vi "OpenNetworkStreamWriter.vi"(6 "connection timeout":i32=-1, 7 "writer buffer size":i32, 8 "error in (no error)":errorcluster, 9 "reader url":string, 10 "writer name":string, 11 "NetworkStreamWriter in":refnum<class "NetworkStreamWriter.lvclass">) -> (0 "error out":errorcluster, 1 "Initialized?":bool, 2 "Writer Endpoint":refnum<k21>, 3 "NetworkStreamWriter out":refnum<class "NetworkStreamWriter.lvclass">)   [LabVIEW 2011, in "NetworkStreamWriter.lvclass"]
doc: "Opens a network stream writer endpoint. This VI persistently tries to open the connection until it is successful or the e-stop is triggered."
uses:
  NetworkStreamWriter.lvclass
  Shared/message.ctl
  NetworkStreamWriter.lvclass/NetworkStreamWriter.ctl
  2-Think/2 Globals/2 Global.vi
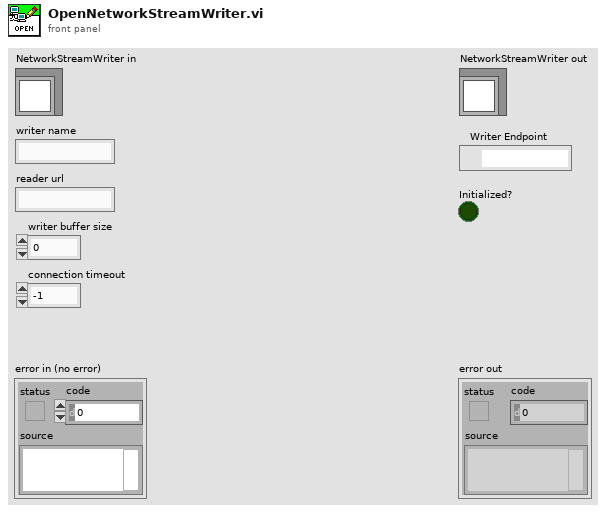
[diagram p1: front panel]
types:
  T1 = typedef "message.ctl" = cluster{"Data":variant, "Time since start (s)":dbl}
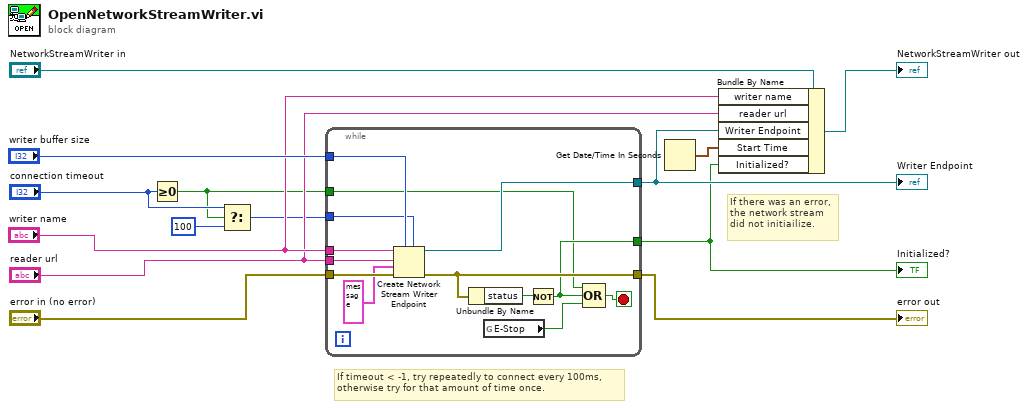
[diagram p0: block diagram]
diagram:
  # "If there was an error,\nthe network stream\ndid not initiailize."
  # "If timeout < -1, try repeatedly to connect every 100ms,\notherwise try for that amount of time once."
  n1 = Greater Or Equal To 0?(x="connection timeout") -> (x >= 0?=w3:bool)
  n2 = Select(t="connection timeout", s=w3, f=100 ("t")) -> (s? t:f=w2:i32)
  n3 = while {
    tunnel: "error in (no error)" -> [w27]
    tunnel: "writer buffer size" -> [w26]
    tunnel: [w22] -> w13
    tunnel: "writer name" -> [w25]
    tunnel: "reader url" -> [w24]
    tunnel: [w21] -> w7
    tunnel: [w18] -> w4
    tunnel: w3 -> [w16]
    tunnel: w2 -> [w15]
    stop <- w19 stop-if-true
    n4 = Create Network Stream Writer Endpoint(5:w15, 7:w26, 8:w27, 9:T1 {"Data"=variant, "Time since start (s)"=0.0} ("variant"), 10:w24, 11:w25) -> (0:w22:errorcluster, 3:w21:refnum<k21>)
    n5 = Unbundle By Name(w22) -> ("status"=w20:bool)
    n6 = global read "2 Global.vi" "E-Stop"() -> (w17:bool)
    n7 = Not(x=w20) -> (.not. x?=w18:bool)
    n8 = Compound Arithmetic op=OR(w16, w18, w17) -> (w19:bool)
  }
  "error out" <- w13
  "Writer Endpoint" <- w7
  "Initialized?" <- w4
  n9 = Get Date/Time In Seconds() -> (seconds since 1Jan1904=w5:timestamp)
  n10 = Bundle By Name(cluster="NetworkStreamWriter in", "writer name"="writer name", "reader url"="reader url", "Writer Endpoint"=w7, "Start Time"=w5, "Initialized?"=w4) -> (→"NetworkStreamWriter out":refnum<class "NetworkStreamWriter.lvclass">)
